vi "Write Class Ref.vi"(8 "error in (no error)":errorcluster, 10 "Class Ref":refnum<vi>, 11 "Identity Writer in":refnum<class "Identity Writer.lvclass">) -> (0 "error out":errorcluster, 3 "Identity Writer out":refnum<class "Identity Writer.lvclass">)   [LabVIEW 2013, in "Identity Writer.lvclass"]
uses:
  Identity Writer.lvclass
  Identity Writer.lvclass/Identity Writer.ctl
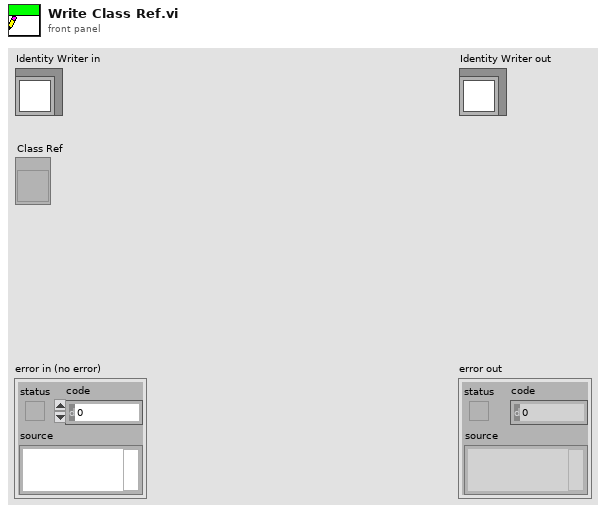
[diagram p1: front panel]
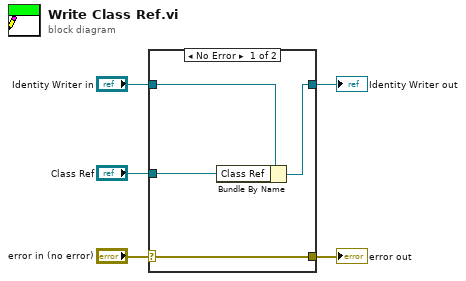
[diagram p0: block diagram]
diagram:
  n1 = case shown="No Error" "error in (no error)" {
    selector: "error in (no error)" -> [w9 w10]
    tunnel: [w9 w10] -> w4
    tunnel: [w7 w11] -> w2
    tunnel: "Identity Writer in" -> [w8 w11]
    tunnel: "Class Ref" -> [w6 _]
    frame No Error {
      n2 = Bundle By Name(cluster=w8, "Class Ref"=w6) -> (w7:refnum<class "Identity Writer.lvclass">)
    }
    frame Error {
    }
  }
  "error out" <- w4
  "Identity Writer out" <- w2
